vi "SpareRelay(SPDT)_encode.vi"(8 "error in (no error)":errorcluster, 10 "data":bool[](array[boolean])=[FALSE, FALSE, FALSE, FALSE, FALSE, FALSE, FALSE, FALSE, FALSE, FALSE, FALSE, FALSE, FALSE, FALSE, FALSE, FALSE, FALSE, FALSE, FALSE, FALSE], 11 "Mem_mapping in":u16[](array[numeric])) -> (0 "error out":errorcluster, 3 "MemMapping Out":u16[](array[numeric]))   [LabVIEW 2018, in "MB Relay.lvlib"]
uses:
  MB Relay.lvlib
panel:
  out "Data":u16[](array[numeric])
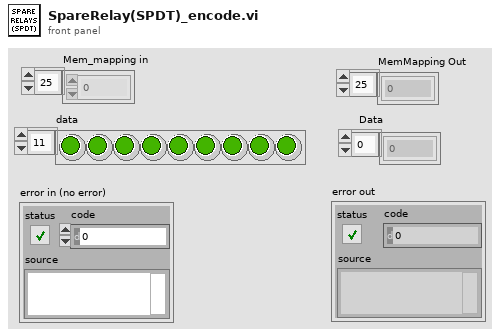
[diagram p1: front panel]
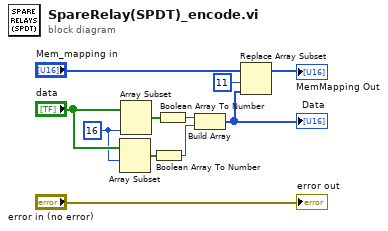
[diagram p0: block diagram]
diagram:
  w9 = 16 ("length")
  n1 = Array Subset(array="data", index=w9) -> (w7:bool[])  [unwired: 1 in]
  n2 = Array Subset(array="data", length=w9) -> (w8:bool[])  [unwired: 1 in]
  n3 = Boolean Array To Number(Boolean array=w7) -> (number=w5:u16)
  n4 = Boolean Array To Number(Boolean array=w8) -> (number=w6:u16)
  n5 = Build Array(w6, w5) -> (w1:u16[])
  "Data" <- w1
  n6 = Replace Array Subset(array="Mem_mapping in", new element=w1, index=11) -> (→"MemMapping Out":u16[])
  "error out" <- "error in (no error)"
